vi "Initialize with copy transmission.vi"(8 "error in (no error)":errorcluster, 9 "unit ID":u8=1, 10 "MB Serial copy":refnum<class "Modbus Master CR.lvclass">, 11 "MB Serial in":refnum<class "Serial.lvclass">) -> (0 "error out":errorcluster, 3 "MB Serial out":refnum<class "Serial.lvclass">)   [LabVIEW 2021, in "Serial.lvclass"]
uses:
  Serial.lvclass
  D:/my_projects/projects/Algorithms/Labview/21/Modbus_v121c/Network Protocol/MB/Modbus Master CR.lvclass
  MB/Modbus Master CR.lvclass
  MB/Modbus Master CR.lvclass/Modbus Master CR.ctl
  MB/ctl/MB timeouts.ctl
  MB Param/MBTCP Param/MBTCP Param.lvclass
  MB Param/MBTCP Param/MBTCP Param.lvclass/MBTCP Param.ctl
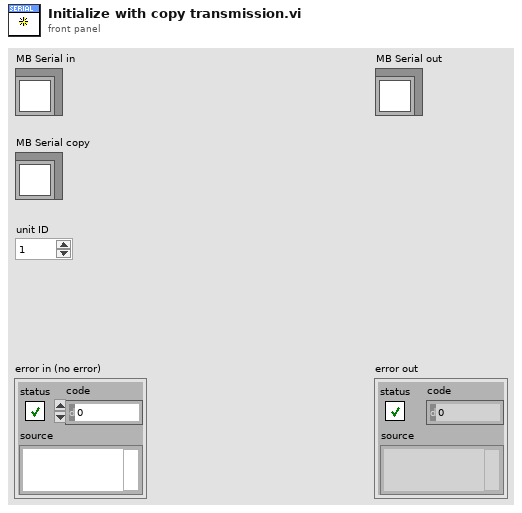
[diagram p1: front panel]
types:
  T1 = typedef "Modbus Master CR.lvclass/MB timeouts.ctl" = cluster{"reconn_timeout":i32, "N attempt max":i32, "t_reset_TTL":i32, "period":i32}
  T2 = typedef "MBParam.lvlib/MBTCP Param.lvclass/timeouts.ctl" = cluster{"conn_timeout":i32, "reconn_timeout":i32, "N attempt max":i32, "t_reset_TTL":i32, "write_timeout":i32, "read_timeout":i32, "period":i32}
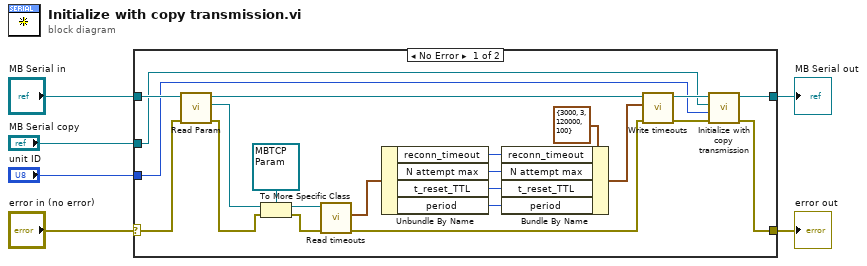
[diagram p0: block diagram]
diagram:
  n1 = case shown="No Error" "error in (no error)" {
    selector: "error in (no error)" -> [w7 w29]
    tunnel: [w11 w29] -> w5
    tunnel: [w12 w30] -> w3
    tunnel: "MB Serial in" -> [w10 w30]
    tunnel: "MB Serial copy" -> [w9 _]
    tunnel: "unit ID" -> [w8 _]
    frame No Error {
      n2 = call "Read Param.vi"("error in (no error)"=w7, "MB_TCP in"=w10) -> ("error out"=w16:errorcluster, "Param"=w17:refnum<class "MB Param.lvclass">, "MB_TCP out"=w18:refnum<class "Serial.lvclass">)  [unwired: 7 in]
      n3 = To More Specific Class(target class=refnum<class "MBTCP Param.lvclass"> refnum ("MBParam.lvlib:MBTCP Param.lvclass"), reference=w17, error in=w16) -> (specific class reference=w26:refnum<class "MBTCP Param.lvclass">, error out=w27:errorcluster)
      n4 = call "Read timeouts.vi"("error in (no error)"=w27, "MBParam in"=w26) -> ("error out"=w15:errorcluster, "timeouts"=w19:T2)  [unwired: 7 in, 1 out]
      n5 = Unbundle By Name(w19) -> ("reconn_timeout"=w24:i32, "N attempt max"=w21:i32, "t_reset_TTL"=w22:i32, "period"=w23:i32)
      n6 = Bundle By Name(cluster=T1 {"reconn_timeout"=3000, "N attempt max"=3, "t_reset_TTL"=120000, "period"=100} ("MB timeouts"), "reconn_timeout"=w24, "N attempt max"=w21, "t_reset_TTL"=w22, "period"=w23) -> (w20:T1)
      n7 = call "Write timeouts.vi"("error in (no error)"=w15, "MB timeouts"=w20, "MB_TCP in"=w18) -> ("error out"=w13:errorcluster, "MB_TCP out"=w14:refnum<class "Serial.lvclass">)  [unwired: 7 in]
      n8 = call-parent "Initialize with copy transmission.vi"("error in (no error)"=w13, "unit ID"=w8, "MB copy"=w9, "MB in"=w14) -> ("error out"=w11:errorcluster, "MB out"=w12:refnum<class "Serial.lvclass">)  [unwired: 6 in]
    }
    frame Error {
    }
  }
  "error out" <- w5
  "MB Serial out" <- w3
